vi "ChooseSwerveCenter.vi"(6 "Defensive Driving Trigger":bool, 8 "Joystick Y":dbl, 9 "Joystick X":dbl) -> (3 "Center Choice":T1(ring))   [LabVIEW 2019]
doc: "***under development***"
uses:
  9a94878a-4914-4fba-839a-7657b048eec0.vi
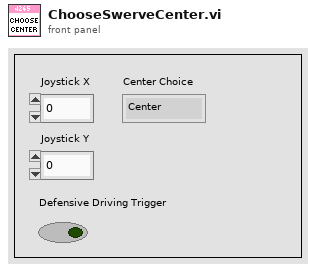
[diagram p1: front panel]
types:
  T1 = enum16{"Center", "Module 0", "Module 1", "Module 2", "Module 3"}
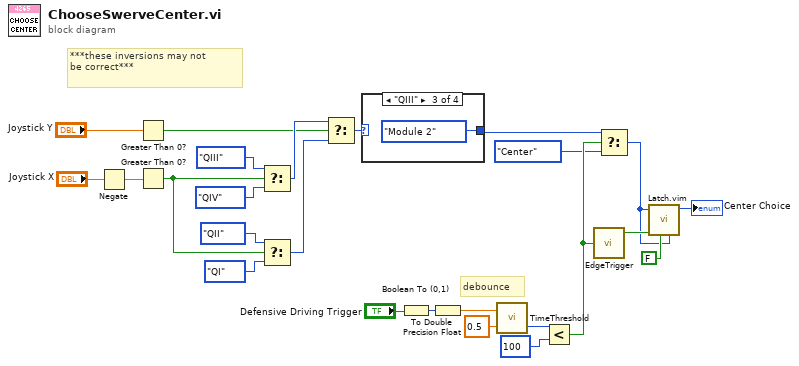
[diagram p0: block diagram]
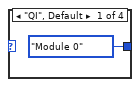
[diagram p2: hidden frame]
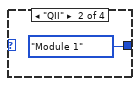
[diagram p3: hidden frame]
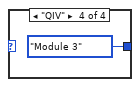
[diagram p4: hidden frame]
diagram:
  # "***these inversions may not\nbe correct***"
  # "debounce"
  n1 = Negate(x="Joystick X") -> (-x=w19:dbl)
  n2 = Greater Than 0?(x="Joystick Y") -> (x > 0?=w22:bool)
  n3 = Greater Than 0?(x=w19) -> (x > 0?=w24:bool)
  n4 = Select(t=enum16{"QI", "QII", "QIII", "QIV"}."QIII", s=w24, f=enum16{"QI", "QII", "QIII", "QIV"}."QIV") -> (s? t:f=w23:enum16{"QI", "QII", "QIII", "QIV"})
  n5 = Select(t=enum16{"QI", "QII", "QIII", "QIV"}."QII", s=w24, f=enum16{"QI", "QII", "QIII", "QIV"}."QI") -> (s? t:f=w25:enum16{"QI", "QII", "QIII", "QIV"})
  n6 = Select(t=w23, s=w22, f=w25) -> (s? t:f=w10:enum16{"QI", "QII", "QIII", "QIV"})
  n7 = case shown="\"QIII\"" w10 {
    tunnel: [T1."Module 0" T1."Module 1" T1."Module 2" T1."Module 3"] -> w3
    frame "QI", Default {
    }
    frame "QII" {
    }
    frame "QIII" {
    }
    frame "QIV" {
    }
  }
  n8 = Boolean To (0,1)(Boolean="Defensive Driving Trigger") -> (0, 1=w14:i16)
  n9 = To Double Precision Float(number=w14) -> (double precision float=w13:dbl)
  n10 = call "TimeThreshold.vi"("Threshold"=0.5, "Current Value"=w13) -> ("Time Below Threshold (ms)"=w12:u32)  [unwired: 1 out]
  n11 = Less?(x=w12, y=u32 100) -> (x < y?=w9:bool)
  n12 = call "EdgeTrigger.vi"("Input Signal"=w9) -> ("Rising Edge Trigger"=w18:bool)  [unwired: 2 out]
  n13 = Select(t=w3, s=w9, f=T1."Center") -> (s? t:f=w2:T1)
  n14 = call "Latch.vim"("Default Value"=w2, "Reset"=FALSE, "Latch Signal"=w18, "Latch Value"=w2) -> ("Latched"=→"Center Choice":T1)  [unwired: 7 in]
